vi "BlockDiagram_SetInputs.vi"(6 "error in":errorcluster, 9 "PythonConverter_BD in":refnum<class "PyConvBD.lvclass">) -> (0 "error out":errorcluster, 3 "PythonConverter_BD out":refnum<class "PyConvBD.lvclass">, 4 "set_inputs":string)   [LabVIEW 2014, in "Raspberry Pi Compatible Compiler for LabVIEW.lvlib" / "PyConvBD.lvclass"]
uses:
  PyConvBD.lvclass
  Parsing/ClassTypeTD.ctl
  PyConvBD.lvclass/PyConvBD.ctl
  VI Interpreter/Classes/ControlTerminal/ControlTerminal.lvclass
  VI Interpreter/Classes/TopLevelDiagram/TopLevelDiagram.lvclass
  Parsing/Python Functions.lvlib
  VI Interpreter/Classes/VI Interpreter/VI Interpreter.lvclass
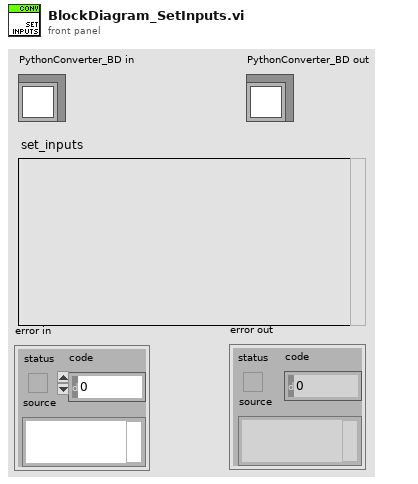
[diagram p1: front panel]
types:
  T1 = typedef "Raspberry Pi Compatible Compiler for LabVIEW.lvlib/Python Functions.lvlib/ClassTypeTD.ctl" = enum16{"class", "function"}
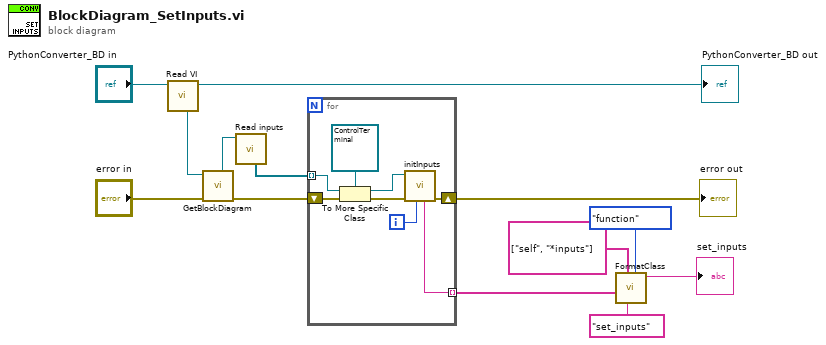
[diagram p0: block diagram]
diagram:
  n1 = call "Read VI.vi"("PythonConverter_BD in"="PythonConverter_BD in") -> ("PythonConverter_BD out"=→"PythonConverter_BD out":refnum<class "PyConvBD.lvclass">, "VI Interpreter"=w6:refnum<class "VI Interpreter.lvclass">)  [unwired: 7 in]
  n2 = call "GetBlockDiagram.vi"("error in"="error in", "VI Interpreter in"=w6) -> ("error out"=w7:errorcluster, "TopLevelDiagram"=w9:refnum<class "TopLevelDiagram.lvclass">)  [unwired: 5 in, 1 out]
  n3 = call-dynamic "Read inputs.vi"("Diagram in"=w9) -> ("inputs"=w8:refnum<class "Terminal.lvclass">[])  [unwired: 7 in, 1 out]
  n4 = for {
    tunnel: w8 -> [w14] mode=indexing
    shift-right: [w21] -> w2
    shift-left: w7 -> [w18]
    tunnel: [w20] -> w11 mode=indexing
    i -> [w19]
    n5 = To More Specific Class(target class=refnum<class "ControlTerminal.lvclass"> refnum ("Control Terminal in"), reference=w14, error in=w18) -> (specific class reference=w16:refnum<class "ControlTerminal.lvclass">, error out=w17:errorcluster)
    n6 = call "initInputs.vi"("index"=w19, "error in"=w17, "Control Terminal in"=w16) -> ("error out"=w21:errorcluster, "initValues"=w20:string)  [unwired: 4 in, 1 out]
  }
  "error out" <- w2
  n7 = call "FormatClass.vi"("type"=ClassTypeTD."function", "name"="set_inputs", "parameters/ancestors"=string[] ["self", "*inputs"], "body"=w11) -> ("python"=→"set_inputs":string)  [unwired: 7 in]
